vi "XML Script - Control (Variant).vi"(0 "x":i32=-1, 1 "y":i32=-1, 2 "out":i32=-1, 3 "conpane index":i32=-1, 4 "type index":i32=-1, 6 "name":string, 8 "indicator?":bool, 9 "prefix (name)":string, 10 "in":i32=-1, 11 "label":string) -> (5 "name (wire source)":string, 7 "XML Script Command - Control":string)   [LabVIEW 2017]
uses:
  <vilib>/_script/XML Scripting/XML Script Attribute.ctl
  <vilib>/_script/XML Scripting/XML Script Tag.ctl
panel:
  # "position"
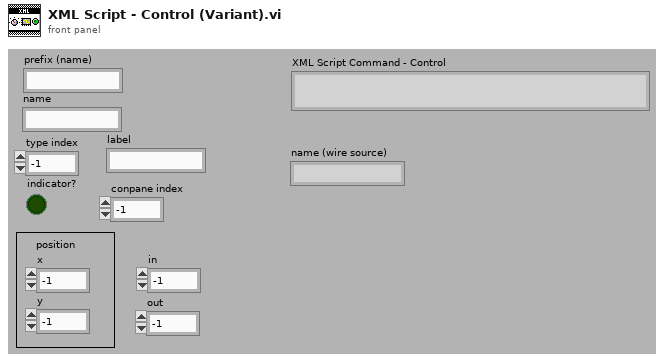
[diagram p1: front panel]
types:
  T1 = typedef "XML Script Attribute.ctl" = enum16{"name", "style", "path", "position", "in", "out", "width", "height", "index", "value", "default", "location", "offset", "typeindex", "size", "source", "destination", "indicator", "type", "controlname", "label", "conpaneidx", "mode", "description", "hasCondTerm", "linkIdentity", "caseselectortype", "concatInputs", "inName", "instantiationpath", "loopCondition", "IndexMode", "formulaInputs", "formulaOutputs", "msnFuncName", "msnIsDynamic", "msnIsODEUserFunction", "ignoreSearchDialog"}
  T2 = typedef "XML Script Tag.ctl" = enum16{"Script", "Function", "SubVI", "GrowableFunction", "Structure", "MultiframeStructure", "Frame", "Tunnel", "ShiftRegister", "Constant", "Control", "Terminal", "Wire", "StaticVIReference", "ControlTerminal", "CompoundArithmetic", "FlatSequence", "FlatSequenceFrame", "MathScriptCallByRef", "BuildArray", "GenericSubVI", "MathScriptNode"}
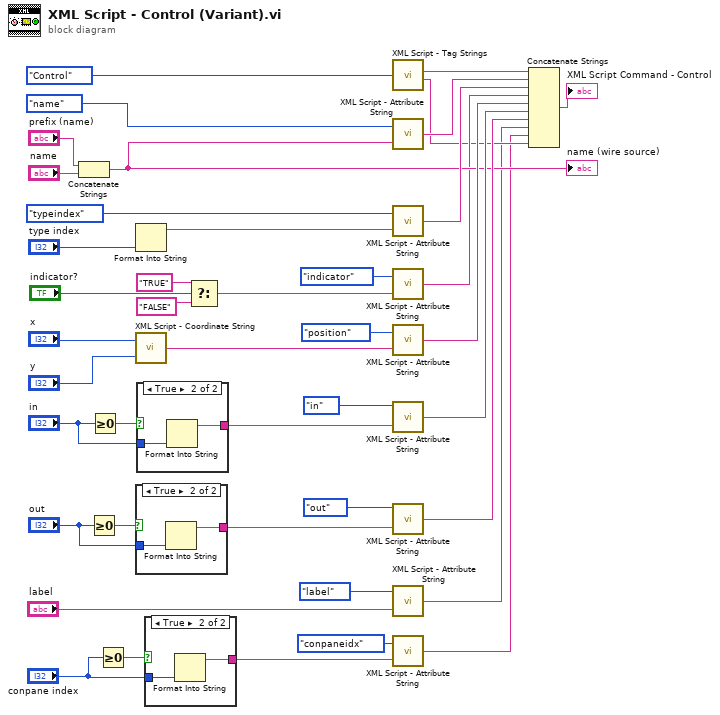
[diagram p0: block diagram]
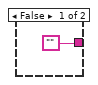
[diagram p2: hidden frame]
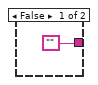
[diagram p3: hidden frame]
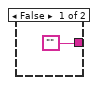
[diagram p4: hidden frame]
diagram:
  n1 = Concatenate Strings("prefix (name)", "name") -> (w18:string)
  "name (wire source)" <- w18
  n2 = Greater Or Equal To 0?(x="out") -> (x >= 0?=w30:bool)
  n3 = Greater Or Equal To 0?(x="in") -> (x >= 0?=w21:bool)
  n4 = Greater Or Equal To 0?(x="conpane index") -> (x >= 0?=w5:bool)
  n5 = Format Into String("type index") -> (resulting string=w24:string)  [unwired: 3 in, 1 out]
  n6 = call <vilib>:"XML Script - Coordinate String.vi"("y"="y", "x"="x") -> ("(x,y)"=w39:string)
  n7 = case shown="True" w30 {
    tunnel: "out" -> [_ w45]
    tunnel: ["" w44] -> w27
    frame False {
    }
    frame True {
      n8 = Format Into String(w45) -> (resulting string=w44:string)  [unwired: 3 in, 1 out]
    }
  }
  n9 = case shown="True" w21 {
    tunnel: "in" -> [_ w48]
    tunnel: ["" w47] -> w23
    frame False {
    }
    frame True {
      n10 = Format Into String(w48) -> (resulting string=w47:string)  [unwired: 3 in, 1 out]
    }
  }
  n11 = case shown="True" w5 {
    tunnel: "conpane index" -> [_ w51]
    tunnel: ["" w50] -> w3
    frame False {
    }
    frame True {
      n12 = Format Into String(w51) -> (resulting string=w50:string)  [unwired: 3 in, 1 out]
    }
  }
  n13 = Select(t="TRUE", s="indicator?", f="FALSE") -> (s? t:f=w12:string)
  n14 = call <vilib>:"XML Script - Tag Strings.vi"("XML Script Tag"=XML_Script_Tag."Control") -> ("XML String - Begin Tag"=w36:string, "XML String - End Tag"=w7:string)  [unwired: 2 in]
  n15 = call <vilib>:"XML Script - Attribute String.vi"("Attribute String"=w18, "XML Script Attribute"=XML_Script_Attribute."name") -> ("XML Script - Attribute String"=w34:string)
  n16 = call <vilib>:"XML Script - Attribute String.vi"("Attribute String"=w24, "XML Script Attribute"=XML_Script_Attribute."typeindex") -> ("XML Script - Attribute String"=w32:string)
  n17 = call <vilib>:"XML Script - Attribute String.vi"("Attribute String"=w12, "XML Script Attribute"=XML_Script_Attribute."indicator") -> ("XML Script - Attribute String"=w10:string)
  n18 = call <vilib>:"XML Script - Attribute String.vi"("Attribute String"=w39, "XML Script Attribute"=XML_Script_Attribute."position") -> ("XML Script - Attribute String"=w31:string)
  n19 = call <vilib>:"XML Script - Attribute String.vi"("Attribute String"=w23, "XML Script Attribute"=XML_Script_Attribute."in") -> ("XML Script - Attribute String"=w19:string)
  n20 = call <vilib>:"XML Script - Attribute String.vi"("Attribute String"=w27, "XML Script Attribute"=XML_Script_Attribute."out") -> ("XML Script - Attribute String"=w26:string)
  n21 = call <vilib>:"XML Script - Attribute String.vi"("Attribute String"="label", "XML Script Attribute"=XML_Script_Attribute."label") -> ("XML Script - Attribute String"=w6:string)
  n22 = call <vilib>:"XML Script - Attribute String.vi"("Attribute String"=w3, "XML Script Attribute"=XML_Script_Attribute."conpaneidx") -> ("XML Script - Attribute String"=w2:string)
  n23 = Concatenate Strings(w36, w34, w32, w10, w31, w19, w26, w6, w2, w7) -> (→"XML Script Command - Control":string)
